vi "GraphTool.vi"() -> ()   [LabVIEW 2014]
uses:
  GrpahTools.ctl
  <vilib>/Utility/miscctls.llb/LVPositionTypeDef.ctl
panel:
  in  "Stop":bool
  in  "Active Channel":u16(ring) items=["Channel 1", "Channel 2"]
  in  "Graph Tools":T1
  in  "Colormap":T2(ring)
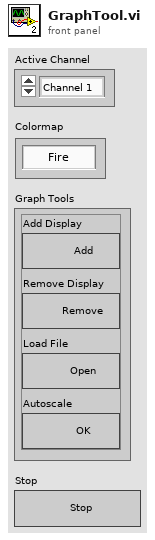
[diagram p1: front panel]
types:
  T1 = typedef "GrpahTools.ctl" = cluster{"Add Display":bool, "Remove Display":bool, "Autoscale":bool, "Load File":bool}
  T2 = enum16{"Fire", "Gray", "Red", "Green", "Blue", "Cyan", "Magenta", "Yellow", "Red-White", "Green-White", "Blue-White", "Glow"}
  T3 = typedef "LVPositionTypeDef.ctl" = cluster{"Left":i32, "Top":i32}
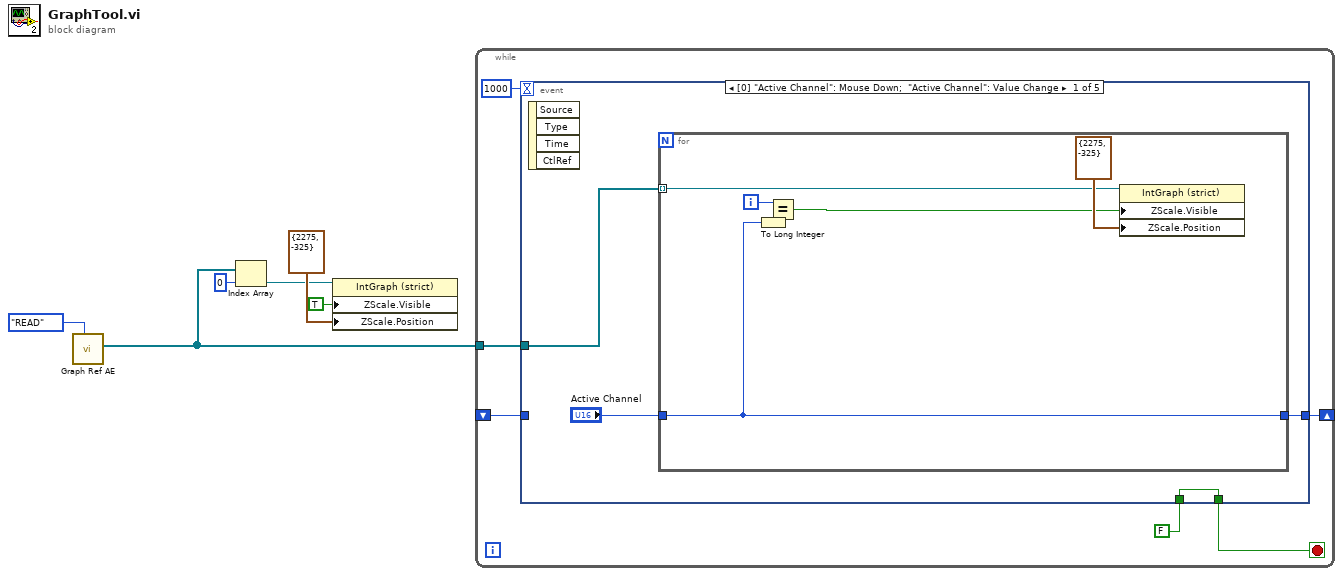
[diagram p0: block diagram]
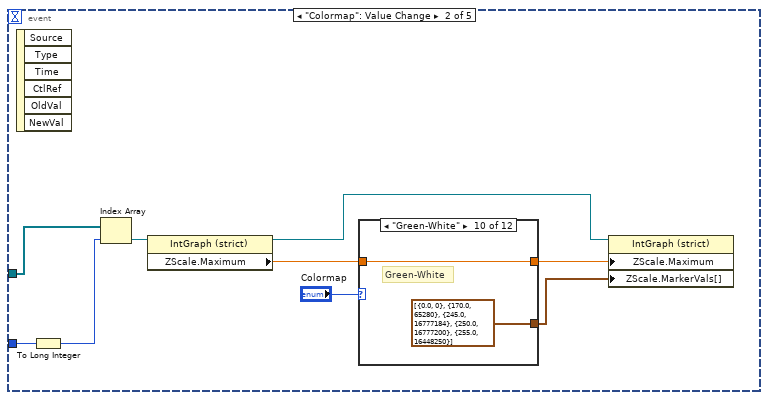
[diagram p2: hidden frame]
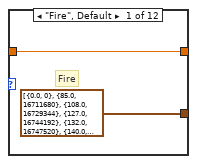
[diagram p3: hidden frame]
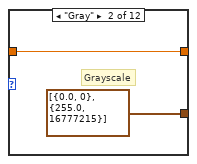
[diagram p4: hidden frame]
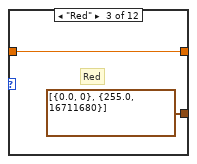
[diagram p5: hidden frame]
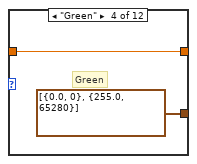
[diagram p6: hidden frame]
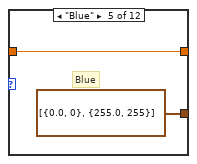
[diagram p7: hidden frame]
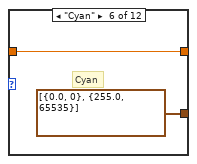
[diagram p8: hidden frame]
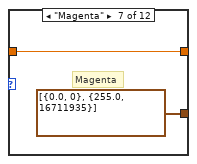
[diagram p9: hidden frame]
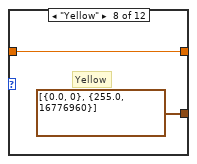
[diagram p10: hidden frame]
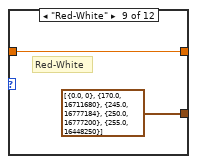
[diagram p11: hidden frame]
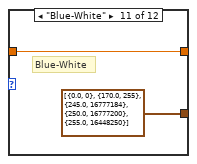
[diagram p12: hidden frame]
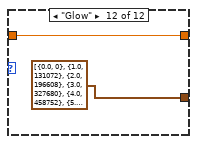
[diagram p13: hidden frame]
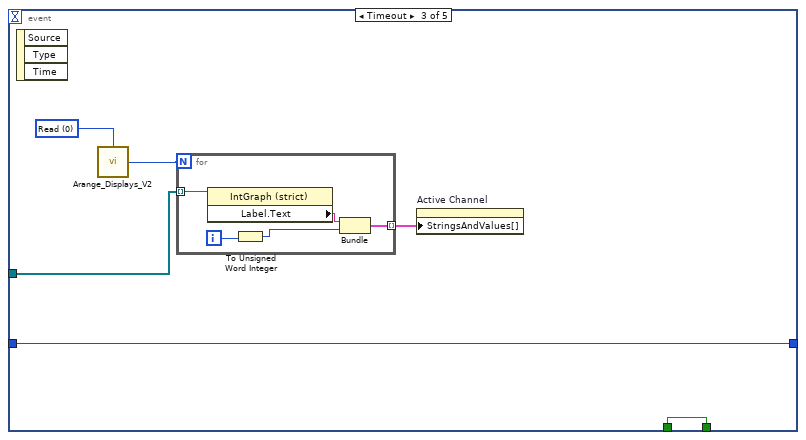
[diagram p14: hidden frame]
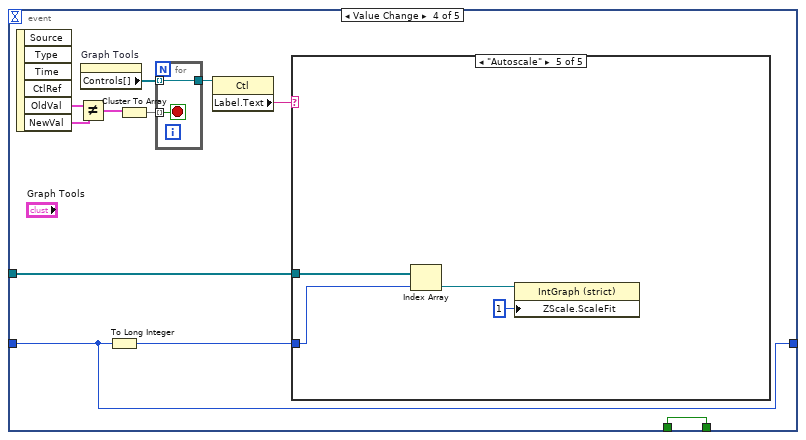
[diagram p15: hidden frame]
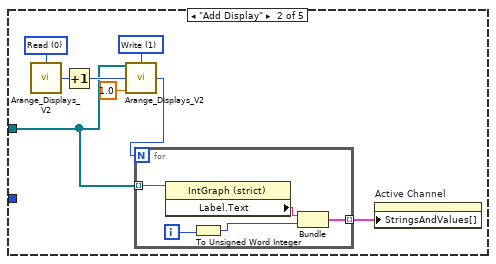
[diagram p17: hidden frame]
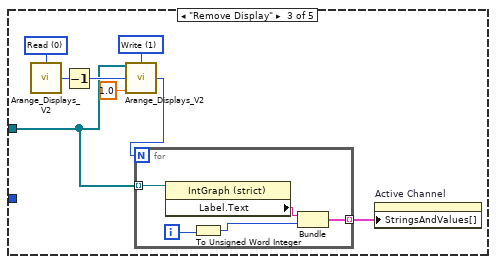
[diagram p18: hidden frame]
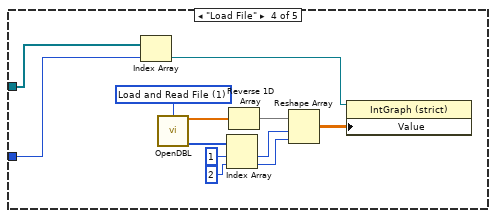
[diagram p19: hidden frame]
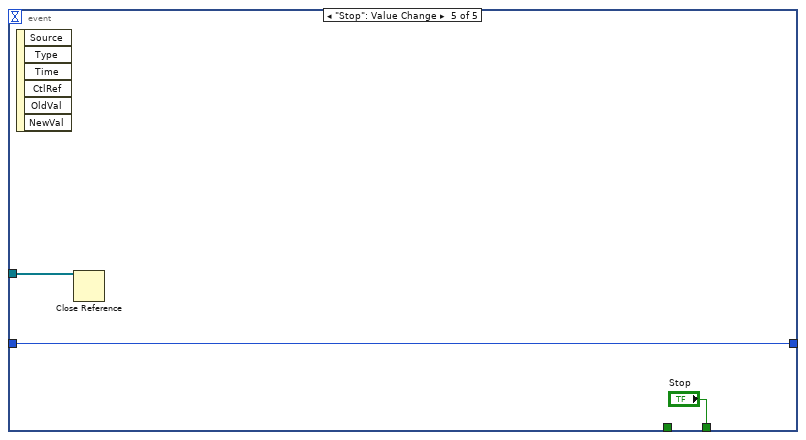
[diagram p20: hidden frame]
diagram:
  n1 = call "Graph Ref AE.vi"("Action"=enum16{"READ", "WRITE"}."READ") -> ("Graph Ref Out"=w4:refnum<vi>[])  [unwired: 10 in]
  n2 = Index Array(array=w4, index=0) -> (element=w3:refnum<vi>)
  n3 = property class="IntGraph (strict)"(reference=w3, "ZScale.Visible"=TRUE ("Z Scale.Visible"), "ZScale.Position"=T3 {"Left"=2275, "Top"=-325} ("Z Scale.Position")) -> ()  [unwired: 1 in, 2 out]
  n4 = while {
    tunnel: w4 -> [w12]
    shift-right: [w9] -> _
    shift-left: _ -> [w8]
    stop <- w11 stop-if-true
    n5 = event shown="[0] \"Active Channel\": Mouse Down;  \"Active Channel\": Value Change" {
      selector: _ -> [_ _ _ _ _]
      dyn-events: _ -> [_ _ _ _ _]
      timeout: 1000 -> [_ _ _ _ _]
      tunnel: w12 -> [w16 w31 w58 w70 w122]
      tunnel: [w15 _ w56 w69 "Stop"] -> w11
      tunnel: FALSE -> [w15 _ w56 w69 _]
      tunnel: [w14 _ w57 w67 w123] -> w9
      tunnel: w8 -> [_ w30 w57 w67 w123]
      event "Active Channel": Mouse Down; "Active Channel": Value Change {
        n6 = event-data() -> ()  [unwired: 1 in, 4 out]
        n7 = for {
          tunnel: w16 -> [w18] mode=indexing
          tunnel: [w17] -> w14
          tunnel: "Active Channel" -> [w17]
          i -> [w21]
          n8 = To Long Integer(number=w17) -> (32bit integer=w20:i32)
          n9 = Equal?(x=w21, y=w20) -> (x = y?=w19:bool)
          n10 = property class="IntGraph (strict)"(reference=w18, "ZScale.Visible"=w19, "ZScale.Position"=T3 {"Left"=2275, "Top"=-325} ("Z Scale.Position")) -> ()  [unwired: 1 in, 2 out]
        }
      }
      event "Colormap": Value Change {
        n11 = event-data() -> ()  [unwired: 1 in, 6 out]
        n12 = To Long Integer(number=w30) -> (32bit integer=w29:i32)
        n13 = Index Array(array=w31, index=w29) -> (element=w27:refnum<vi>)
        n14 = property class="IntGraph (strict)"(reference=w27) -> (reference out=w25:refnum<vi>, "ZScale.Maximum"=w26:dbl)  [unwired: 1 in, 1 out]
        n15 = case shown="\"Green-White\"" "Colormap" {
          tunnel: [cluster{dbl, u32}[] [{0.0, 0}, {85.0, 16711680}, {108.0, 16729344}, {127.0, 16744192}, {132.0, 16747520}, {140.0, 16753920}, {157.0, 16766720}, {170.0, 16776960}, {245.0, 16777184}, {250.0, 16777200}, {255.0, 16777215}] ("Z Scale.Marker Values[]") cluster{dbl, u32}[] [{0.0, 0}, {255.0, 16777215}] ("Z Scale.Marker Values[]") cluster{dbl, u32}[] [{0.0, 0}, {255.0, 16711680}] ("Z Scale.Marker Values[]") cluster{dbl, u32}[] [{0.0, 0}, {255.0, 65280}] ("Z Scale.Marker Values[]") cluster{dbl, u32}[] [{0.0, 0}, {255.0, 255}] ("Z Scale.Marker Values[]") cluster{dbl, u32}[] [{0.0, 0}, {255.0, 65535}] ("Z Scale.Marker Values[]") cluster{dbl, u32}[] [{0.0, 0}, {255.0, 16711935}] ("Z Scale.Marker Values[]") cluster{dbl, u32}[] [{0.0, 0}, {255.0, 16776960}] ("Z Scale.Marker Values[]") cluster{dbl, u32}[] [{0.0, 0}, {170.0, 16711680}, {245.0, 16777184}, {250.0, 16777200}, {255.0, 16448250}] ("Z Scale.Marker Values[]") cluster{dbl, u32}[] [{0.0, 0}, {170.0, 65280}, {245.0, 16777184}, {250.0, 16777200}, {255.0, 16448250}] ("Z Scale.Marker Values[]") cluster{dbl, u32}[] [{0.0, 0}, {170.0, 255}, {245.0, 16777184}, {250.0, 16777200}, {255.0, 16448250}] ("Z Scale.Marker Values[]") cluster{dbl, u32}[] [{0.0, 0}, {1.0, 131072}, {2.0, 196608}, {3.0, 327680}, {4.0, 458752}, {5.0, 589824}, {6.0, 720896}, {7.0, 851971}, {8.0, 983043}, {9.0, 1114115}, {10.0, 1245187}, {11.0, 1376259}, {12.0, 1507331}, {13.0, 1638403}, {14.0, 1769475}, {15.0, 1769479}, {16.0, 2031623}, {17.0, 2162695}, {18.0, 2293767}, {19.0, 2424839}, {20.0, 2555911}, {21.0, 2686983}, {22.0, 2818055}, {23.0, 2949127}, {24.0, 3080203}, {25.0, 3211275}, {26.0, 3342347}, {27.0, 3473419}, {28.0, 3604491}, {29.0, 3735563}, {30.0, 3866635}, {31.0, 3867403}, {32.0, 4129547}, {33.0, 4260619}, {34.0, 4391691}, {35.0, 4522763}, {36.0, 4653839}, {37.0, 4784911}, {38.0, 4915983}, {39.0, 5178127}, {40.0, 5309199}, {41.0, 5440271}, {42.0, 5571343}, {43.0, 5702415}, {44.0, 5703439}, {45.0, 5965583}, {46.0, 6096655}, {47.0, 6227727}, {48.0, 6358799}, {49.0, 6489871}, {50.0, 6620943}, {51.0, 6752015}, {52.0, 6883087}, {53.0, 7015183}, {54.0, 7146255}, {55.0, 7277327}, {56.0, 7408399}, {57.0, 7539471}, {58.0, 7670543}, {59.0, 7801615}, {60.0, 8063759}, {61.0, 8194831}, {62.0, 8326927}, {63.0, 8457999}, {64.0, 8589075}, {65.0, 8720147}, {66.0, 8851219}, {67.0, 8982291}, {68.0, 9113363}, {69.0, 9114387}, {70.0, 9376531}, {71.0, 9507603}, {72.0, 9638675}, {73.0, 9769747}, {74.0, 9901843}, {75.0, 10032915}, {76.0, 10163987}, {77.0, 10229523}, {78.0, 10295059}, {79.0, 10427155}, {80.0, 10558227}, {81.0, 10689299}, {82.0, 10820371}, {83.0, 10886931}, {84.0, 10952467}, {85.0, 11083539}, {86.0, 11214611}, {87.0, 11215635}, {88.0, 11477779}, {89.0, 11543315}, {90.0, 11608851}, {91.0, 11740947}, {92.0, 11806483}, {93.0, 11872019}, {94.0, 12004115}, {95.0, 12135187}, {96.0, 12266259}, {97.0, 12267283}, {98.0, 12398355}, {99.0, 12529427}, {100.0, 12530451}, {101.0, 12595987}, {102.0, 12530451}, {103.0, 12793619}, {104.0, 12794131}, {105.0, 12794643}, {106.0, 13056787}, {107.0, 13057299}, {108.0, 13057811}, {109.0, 13188883}, {110.0, 13320979}, {111.0, 13386515}, {112.0, 13452563}, {113.0, 13584147}, {114.0, 13584659}, {115.0, 13585171}, {116.0, 13585683}, {117.0, 13717267}, {118.0, 13848339}, {119.0, 13849363}, {120.0, 13849875}, {121.0, 13850387}, {122.0, 13981459}, {123.0, 14113555}, {124.0, 14114067}, {125.0, 14114579}, {126.0, 14115091}, {127.0, 14246675}, {128.0, 14377747}, {129.0, 14378771}, {130.0, 14379283}, {131.0, 14379539}, {132.0, 14379795}, {133.0, 14380819}, {134.0, 14511891}, {135.0, 14643987}, {136.0, 14644503}, {137.0, 14645015}, {138.0, 14645527}, {139.0, 14646039}, {140.0, 14646551}, {141.0, 14778135}, {142.0, 14909207}, {143.0, 14910231}, {144.0, 14910747}, {145.0, 14911259}, {146.0, 14911771}, {147.0, 14912283}, {148.0, 14912797}, {149.0, 15044383}, {150.0, 15175455}, {151.0, 15175967}, {152.0, 15176479}, {153.0, 15176991}, {154.0, 15177507}, {155.0, 15178019}, {156.0, 15178531}, {157.0, 15310115}, {158.0, 15441701}, {159.0, 15441959}, {160.0, 15442215}, {161.0, 15442727}, {162.0, 15443243}, {163.0, 15443755}, {164.0, 15444269}, {165.0, 15444783}, {166.0, 15444783}, {167.0, 15576367}, {168.0, 15707953}, {169.0, 15708467}, {170.0, 15708979}, {171.0, 15708981}, {172.0, 15708983}, {173.0, 15710011}, {174.0, 15710523}, {175.0, 15711037}, {176.0, 15711039}, {177.0, 15711553}, {178.0, 15843139}, {179.0, 15974213}, {180.0, 15974215}, {181.0, 15974217}, {182.0, 15974219}, {183.0, 15975755}, {184.0, 15976271}, {185.0, 15976785}, {186.0, 15977299}, {187.0, 15977301}, {188.0, 15977815}, {189.0, 15978327}, {190.0, 15978331}, {191.0, 16109917}, {192.0, 16241503}, {193.0, 16241505}, {194.0, 16242019}, {195.0, 16242535}, {196.0, 16242537}, {197.0, 16242539}, {198.0, 16243563}, {199.0, 16243567}, {200.0, 16244081}, {201.0, 16244595}, {202.0, 16244599}, {203.0, 16244601}, {204.0, 16244603}, {205.0, 16245627}, {206.0, 16245631}, {207.0, 16245633}, {208.0, 16246147}, {209.0, 16246663}, {210.0, 16377735}, {211.0, 16508811}, {212.0, 16508815}, {213.0, 16509839}, {214.0, 16509843}, {215.0, 16509845}, {216.0, 16509847}, {217.0, 16510361}, {218.0, 16510875}, {219.0, 16510879}, {220.0, 16510881}, {221.0, 16510883}, {222.0, 16511399}, {223.0, 16511911}, {224.0, 16511915}, {225.0, 16511917}, {226.0, 16511919}, {227.0, 16511923}, {228.0, 16512437}, {229.0, 16512951}, {230.0, 16512955}, {231.0, 16512957}, {232.0, 16512959}, {233.0, 16512961}, {234.0, 16512963}, {235.0, 16512967}, {236.0, 16513481}, {237.0, 16513995}, {238.0, 16513999}, {239.0, 16514001}, {240.0, 16514003}, {241.0, 16514005}, {242.0, 16514007}, {243.0, 16514011}, {244.0, 16514013}, {245.0, 16514015}, {246.0, 16514019}, {247.0, 16514021}, {248.0, 16514023}, {249.0, 16514027}, {250.0, 16514029}, {251.0, 16514031}, {252.0, 16514035}, {253.0, 16514037}, {254.0, 16514039}, {255.0, 16514043}] ("Z Scale.Marker Values[]")] -> w23
          tunnel: [w32 w34 w36 w38 w40 w42 w44 w46 w48 w50 w52 w54] -> w24
          tunnel: w26 -> [w32 w34 w36 w38 w40 w42 w44 w46 w48 w50 w52 w54]
          frame "Fire", Default {
            # "Fire"
          }
          frame "Gray" {
            # "Grayscale"
          }
          frame "Red" {
            # "Red"
          }
          frame "Green" {
            # "Green"
          }
          frame "Blue" {
            # "Blue"
          }
          frame "Cyan" {
            # "Cyan"
          }
          frame "Magenta" {
            # "Magenta"
          }
          frame "Yellow" {
            # "Yellow"
          }
          frame "Red-White" {
            # "Red-White"
          }
          frame "Green-White" {
            # "Green-White"
          }
          frame "Blue-White" {
            # "Blue-White"
          }
          frame "Glow" {
          }
        }
        n16 = property class="IntGraph (strict)"(reference=w25, "ZScale.Maximum"=w24, "ZScale.MarkerVals[]"=w23) -> ()  [unwired: 1 in, 2 out]
      }
      event Timeout {
        w59 = u16 0 items=["Read", "Write"] ("Action")
        n17 = event-data() -> ()  [unwired: 1 in, 3 out]
        n18 = call "Arange_Displays_V2.vi"("Action"=w59) -> ("Number of Channels OUT"=w61:i32)  [unwired: 14 in]
        n19 = for {
          N: w61 -> [_]
          tunnel: w58 -> [w66] mode=indexing
          tunnel: [w62] -> w60 mode=indexing
          i -> [w65]
          n20 = property class="IntGraph (strict)"(reference=w66) -> ("Label.Text"=w64:string)  [unwired: 1 in, 2 out]
          n21 = To Unsigned Word Integer(number=w65) -> (unsigned 16bit integer=w63:u16)
          n22 = Bundle("Label.Text"=w64, w63) -> (w62:cluster{"Label.Text":string, u16})  [unwired: 1 in]
        }
        n23 = property on="Active Channel" class="Ring (strict)"("StringsAndValues[]"=w60) -> ()  [unwired: 2 in, 2 out]
      }
      event Value Change {
        n24 = event-data() -> ("OldVal"=w77:T1, "NewVal"=w76:T1)  [unwired: 1 in, 4 out]
        n25 = Not Equal?(x=w77, y=w76) -> (x != y?=w75:T1)
        n26 = property on="Graph Tools" class="Clust"() -> ("Controls[]"=w73:refnum<vi>[])  [unwired: 2 in, 2 out]
        n27 = To Long Integer(number=w67) -> (32bit integer=w68:i32)
        n28 = Cluster To Array(cluster=w75) -> (array=w74:bool[])
        n29 = for {
          tunnel: w74 -> [w121] mode=indexing
          tunnel: w73 -> [w120] mode=indexing
          tunnel: [w120] -> w72
          stop <- w121 stop-if-true
        }
        n30 = property class="Ctl"(reference=w72) -> ("Label.Text"=w71:string)  [unwired: 1 in, 2 out]
        n31 = case shown="\"Autoscale\"" w71 {
          tunnel: w70 -> [_ w78 w91 w106 w118]
          tunnel: w68 -> [_ _ _ w105 w119]
          frame "False", Default {
          }
          frame "Add Display" {
            w81 = u16 0 items=["Read", "Write"] ("Action")
            w85 = u16 1 items=["Read", "Write"] ("Action")
            n32 = call "Arange_Displays_V2.vi"("Action"=w81) -> ("Number of Channels OUT"=w82:i32)  [unwired: 14 in]
            n33 = Increment(x=w82) -> (x+1=w84:i32)
            n34 = call "Arange_Displays_V2.vi"("Display References"=w78, "Action"=w85, "Number of Channels"=w84, "Aspect Ratio (h/w)"=1.0) -> ("Number of Channels OUT"=w79:i32)  [unwired: 11 in]
            n35 = for {
              N: w79 -> [_]
              tunnel: w78 -> [w90] mode=indexing
              tunnel: [w86] -> w80 mode=indexing
              i -> [w89]
              n36 = property class="IntGraph (strict)"(reference=w90) -> ("Label.Text"=w88:string)  [unwired: 1 in, 2 out]
              n37 = To Unsigned Word Integer(number=w89) -> (unsigned 16bit integer=w87:u16)
              n38 = Bundle("Label.Text"=w88, w87) -> (w86:cluster{"Label.Text":string, u16})  [unwired: 1 in]
            }
            n39 = property on="Active Channel" class="Ring (strict)"("StringsAndValues[]"=w80) -> ()  [unwired: 2 in, 2 out]
          }
          frame "Remove Display" {
            w94 = u16 0 items=["Read", "Write"] ("Action")
            w98 = u16 1 items=["Read", "Write"] ("Action")
            n40 = call "Arange_Displays_V2.vi"("Action"=w94) -> ("Number of Channels OUT"=w95:i32)  [unwired: 14 in]
            n41 = Decrement(x=w95) -> (x-1=w97:i32)
            n42 = call "Arange_Displays_V2.vi"("Display References"=w91, "Action"=w98, "Number of Channels"=w97, "Aspect Ratio (h/w)"=1.0) -> ("Number of Channels OUT"=w92:i32)  [unwired: 11 in]
            n43 = for {
              N: w92 -> [_]
              tunnel: w91 -> [w103] mode=indexing
              tunnel: [w99] -> w93 mode=indexing
              i -> [w102]
              n44 = property class="IntGraph (strict)"(reference=w103) -> ("Label.Text"=w101:string)  [unwired: 1 in, 2 out]
              n45 = To Unsigned Word Integer(number=w102) -> (unsigned 16bit integer=w100:u16)
              n46 = Bundle("Label.Text"=w101, w100) -> (w99:cluster{"Label.Text":string, u16})  [unwired: 1 in]
            }
            n47 = property on="Active Channel" class="Ring (strict)"("StringsAndValues[]"=w93) -> ()  [unwired: 2 in, 2 out]
          }
          frame "Load File" {
            w107 = u16 1 items=["Get Image", "Load and Read File"] ("Action")
            n48 = Index Array(array=w106, index=w105) -> (element=w104:refnum<vi>)
            n49 = call "OpenDBL.vi"("Action"=w107) -> ("Image"=w108:sgl[], "Dimensions (Z, Y, X, t)"=w109:i32[])  [unwired: 12 in, 1 out]
            n50 = Index Array(array=w109, index #1=1 ("index"), index #2=2 ("index")) -> (element #1=w112:i32, element #2=w113:i32)
            n51 = Reverse 1D Array(array=w108) -> (reversed array=w114:sgl[])
            n52 = Reshape Array(w114, w112, w113) -> (w115:sgl[][])
            n53 = property class="IntGraph (strict)"(reference=w104, "Value"=w115) -> ()  [unwired: 1 in, 2 out]
          }
          frame "Autoscale" {
            n54 = Index Array(array=w118, index=w119) -> (element=w117:refnum<vi>)
            n55 = property class="IntGraph (strict)"(reference=w117, "ZScale.ScaleFit"=u8 1 ("Z Scale.Scale Fit")) -> ()  [unwired: 1 in, 2 out]
          }
        }
      }
      event "Stop": Value Change {
        n56 = event-data() -> ()  [unwired: 1 in, 6 out]
        n57 = Close Reference(reference=w122) -> ()  [unwired: 1 in, 1 out]
      }
    }
  }
